vi "Chart-Start Move Span.vi"(7 "VI reference (current VI)":refnum<vi>, 8 "error in (no error)":errorcluster, 10 "Coords":T2, 11 "XY Graph Ref In":refnum<vi>) -> (0 "error out":errorcluster, 2 "Information":T1, 3 "XY Graph Ref Out":refnum<vi>)   [LabVIEW 2020]
uses:
  <vilib>/Utility/miscctls.llb/LVPoint32TypeDef.ctl
  <vilib>/Utility/cursorutil.llb/Set Cursor (Icon Pict).vi
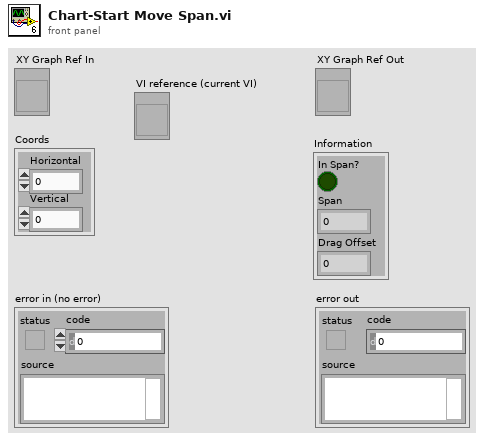
[diagram p1: front panel]
types:
  T1 = cluster{"In Span?":bool, "Span":dbl, "Drag Offset":dbl}
  T2 = typedef "LVPoint32TypeDef.ctl" = cluster{"Horizontal":i32, "Vertical":i32}
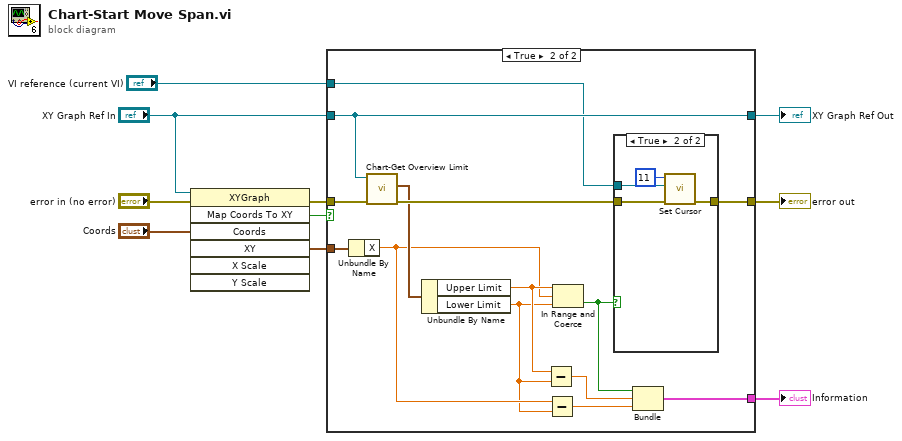
[diagram p0: block diagram]
diagram:
  n1 = invoke on="Invoke Node" class="XYGraph" method="Map Coords To XY"(reference="XY Graph Ref In", error in="error in (no error)", "Coords"="Coords") -> (error out=w6:errorcluster, "Map Coords To XY"=w8:bool, "XY"=w7:cluster{"X":dbl, "Y":dbl})  [unwired: 4 in, 4 out]
  n2 = case shown="True" w8 {
    tunnel: w7 -> [_ w21]
    tunnel: w6 -> [w12 w26]
    tunnel: "XY Graph Ref In" -> [w11 w25]
    tunnel: [w11 w25] -> w3
    tunnel: [w12 w23] -> w4
    tunnel: "VI reference (current VI)" -> [_ w22]
    tunnel: [_ w13] -> w1
    frame False {
    }
    frame True {
      n3 = Unbundle By Name(w21) -> ("X"=w18:dbl)
      n4 = call "Chart-Get Overview Limit.vi"("error in"=w26, "Overview Refnum In"=w25) -> ("error out"=w24:errorcluster, "Limit"=w20:cluster{"Lower Limit":dbl, "Upper Limit":dbl})  [unwired: 7 in, 1 out]
      n5 = Unbundle By Name(w20) -> ("Upper Limit"=w19:dbl, "Lower Limit"=w17:dbl)
      n6 = Subtract(x=w19, y=w17) -> (x-y=w15:dbl)
      n7 = Subtract(x=w18, y=w17) -> (x-y=w16:dbl)
      n8 = In Range and Coerce(upper limit=w19, x=w18, lower limit=w17) -> (In Range?=w14:bool)  [unwired: 1 out]
      n9 = case shown="True" w14 {
        tunnel: w24 -> [w27 w31]
        tunnel: [w27 w29] -> w23
        tunnel: w22 -> [_ w28]
        frame False {
        }
        frame True {
          n10 = call-poly <vilib>:"Set Cursor.vi"("error in (no error)"=w31, "VI reference (current VI)"=w28, "icon"=u16 11) -> ("error out"=w29:errorcluster)  [unwired: 7 in, 1 out]
        }
      }
      n11 = Bundle(w14, w15, w16) -> (w13:cluster{bool, dbl, dbl})  [unwired: 1 in]
    }
  }
  "error out" <- w4
  "XY Graph Ref Out" <- w3
  "Information" <- w1
